vi "Assignment 2.vi"() -> ()   [LabVIEW 2023]
panel:
  in  "Cluster":T1
  out "Student Grade":dbl[](array[numeric])
  in  "stop":bool
  out "average grade":dbl
  out "name":string[](array[string])
  out "NumberofStudents":i32
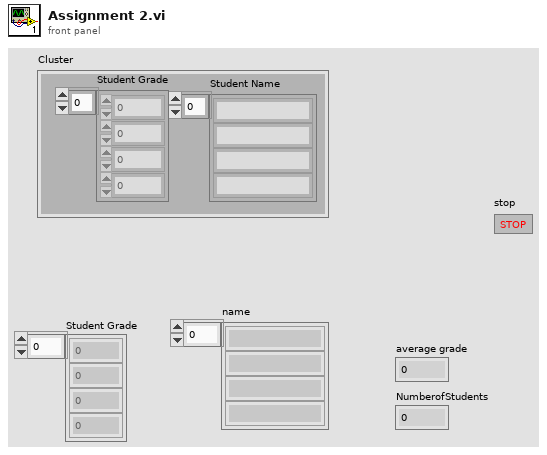
[diagram p1: front panel]
types:
  T1 = cluster{"Student Name":string[], "Student Grade":dbl[]}
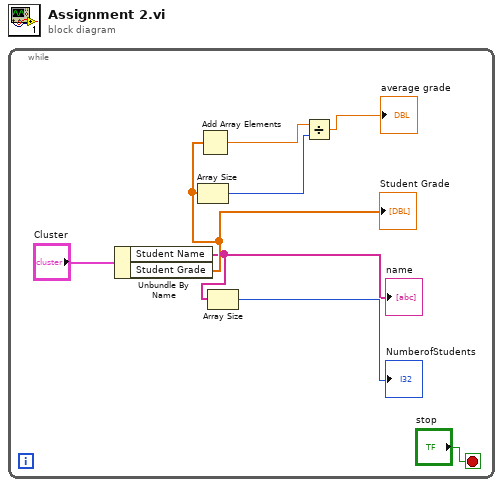
[diagram p0: block diagram]
diagram:
  n1 = while {
    stop <- "stop" stop-if-true
    n2 = Unbundle By Name("Cluster") -> ("Student Name"=w1:string[], "Student Grade"=w2:dbl[])
    "name" <- w1
    "Student Grade" <- w2
    n3 = Array Size(array=w2) -> (size(s)=w6:i32)
    n4 = Add Array Elements(numeric array=w2) -> (sum=w7:dbl)
    n5 = Array Size(array=w1) -> (size(s)=→"NumberofStudents":i32)
    n6 = Divide(x=w7, y=w6) -> (x/y=→"average grade":dbl)
  }
